vi "DSF.Transceiver.GE Reflective Memory.Get Transfer Group Parameters.vi"(11 "GE Reflective Memory in":refnum<class "DSF.Transceiver.GE Reflective Memory.lvclass">) -> (2 "Transfer Group Parameters":T1[](array[typedef]), 3 "GE Reflective Memory out":refnum<class "DSF.Transceiver.GE Reflective Memory.lvclass">)   [LabVIEW 2017, in "DSF.Transceiver.GE Reflective Memory.lvlib" / "DSF.Transceiver.GE Reflective Memory.lvclass"]
uses:
  DSF.Transceiver.GE Reflective Memory.lvclass
  DSF.Transceiver.GE Reflective Memory.Transfer Group Parameters.ctl
  DSF.Transceiver.GE Reflective Memory.lvclass/DSF.Transceiver.GE Reflective Memory.ctl
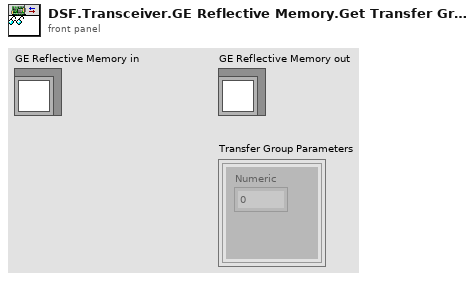
[diagram p1: front panel]
types:
  T1 = typedef "DSF.Transceiver.GE Reflective Memory.lvlib/DSF.Transceiver.GE Reflective Memory.lvclass/DSF.Transceiver.GE Reflective Memory.Transfer Group Parameters.ctl" = cluster{"Numeric":dbl}
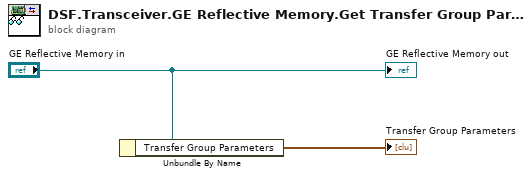
[diagram p0: block diagram]
diagram:
  n1 = Unbundle By Name("GE Reflective Memory in") -> ("Transfer Group Parameters"=→"Transfer Group Parameters":T1[])
  "GE Reflective Memory out" <- "GE Reflective Memory in"
